vi "read_all_waveform_data.vi"(2 "N":i32, 3 "path":string) -> (0 "dt":dbl[](array[numeric]), 1 "data":dbl[](array[numeric]))   [LabVIEW 2022 SP3]
uses:
  <vilib>/Waveform/WDTFileIO.llb/Read Waveform from File.vi
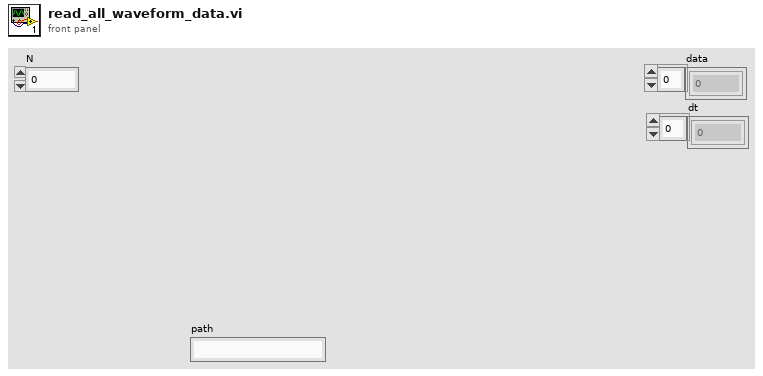
[diagram p1: front panel]
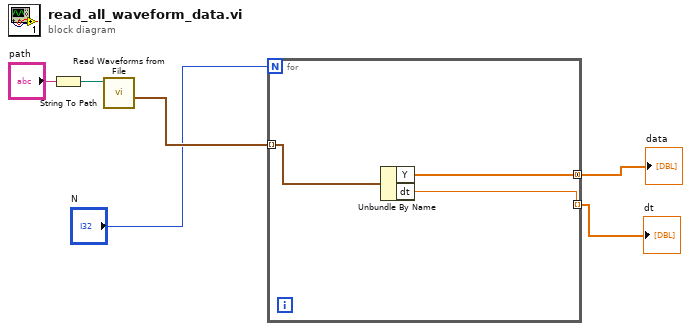
[diagram p0: block diagram]
diagram:
  n1 = String To Path(string="path") -> (path=w6:path)
  n2 = call-poly <vilib>:"Read Waveforms from File.vi"("file path (dialog if empty)"=w6) -> ("all waveforms in record"=w4:waveform(dbl)[])  [unwired: 5 in, 3 out]
  n3 = for {
    N: "N" -> [_]
    tunnel: w4 -> [w9] mode=indexing
    tunnel: [w8] -> w3 mode=concatenating
    tunnel: [w7] -> w2 mode=indexing
    n4 = Unbundle By Name(w9) -> ("Y"=w8:dbl[], "dt"=w7:dbl)
  }
  "data" <- w3
  "dt" <- w2
